vi "fill_in_error_info.vi"(8 "error in (no error)":errorcluster, 10 "path in":path=path "D:/Program Files (x86)/TOSUN/TSMaster/bin/TSMaster.dll", 11 "ACode":i32=81) -> (0 "error out":errorcluster)   [LabVIEW 2014]
doc: "Form fault descriptions into error clusters."
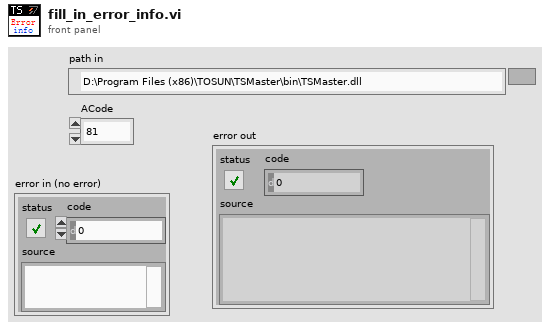
[diagram p1: front panel]
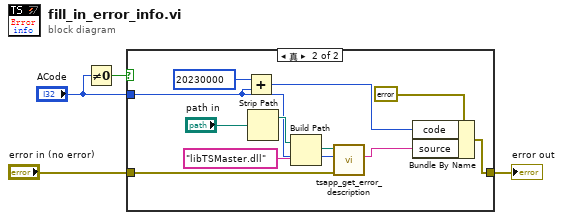
[diagram p0: block diagram]
diagram:
  n1 = Not Equal To 0?(x="ACode") -> (x != 0?=w1:bool)
  n2 = case shown="真" w1 {
    tunnel: "ACode" -> [_ w7]
    tunnel: "error in (no error)" -> [w5 w16]
    tunnel: [w5 w12] -> w4
    frame False {
    }
    frame True {
      n3 = Add(x=20230000 ("error code (0)"), y=w7) -> (x+y=w13:i32)
      n4 = Strip Path(path="path in") -> (stripped path=w11:path)  [unwired: 1 out]
      n5 = Build Path(base path=w11, name or relative path="libTSMaster.dll") -> (appended path=w8:path)
      n6 = call "tsapp_get_error_description.vi"("error in"=w16, "ACount"=w7, "路径输入"=w8) -> ("ErrDes"=w6:string)  [unwired: 6 in, 2 out]
      n7 = Bundle By Name(cluster=errorcluster {"status"=TRUE, "code"=0, "source"=""} ("error constant"), "code"=w13, "source"=w6) -> (w12:errorcluster)
    }
  }
  "error out" <- w4
